vi "ShowRange.Calc.vi"(6 "X-axis devision":i32=1 min=1 max=512, 7 "Current Grating Density":enum16{"150", "300", "600", "1200", "1800"}(ring)=enum."600" caption="Grating Density", 8 "Central Wavelength":dbl=600.0 format="%.2f") -> (0 "meV (Max)":dbl=2170.4007572687524 format="%.2f", 1 "X-axis":dbl[](array[numeric])=[571.2504622529284, 585.6489231225254, 600.0000000000001, 614.300024178551, 628.5453659653462] format="%.4f", 2 "meV (Min)":dbl=1972.5583911666886 format="%.2f", 3 "nm (Max)":dbl=628.5453659653462 format="%.4f", 5 "nm (Min)":dbl=571.2504622529284 format="%.4f")   [LabVIEW 2019]
panel:
  in  "Unit":u16(ring) items=["nm", "cm-1", "meV"]
  out "nm (delta)":dbl=57.29490371241775 format="%.4f"
  out "cm-1 (delta)":dbl=1595.705715333208 format="%.2f"
  out "meV (delta)":dbl=197.8423661020638 format="%.2f"
  out "cm-1 (Max)":dbl=17505.45629418217 format="%.2f"
  out "cm-1 (Min)":dbl=15909.750578848963 format="%.2f"
  out "Detector Pixel Distance":dbl=27.0 format="%.2f"
  out "beta":dbl=0.03851514953863218 format="%.2f"
  out "alpha":dbl=21.141484850461367 format="%.2f"
  out "Spectrometer Mirror angle":dbl=21.18 format="%.2f"
  out "Spectrometer Focal length":dbl=750.0 format="%.1f"
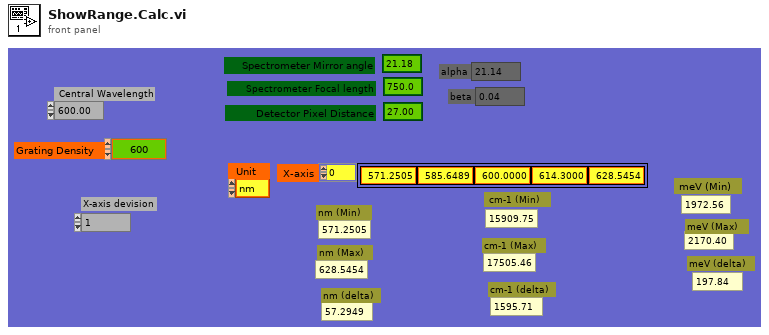
[diagram p1: front panel]
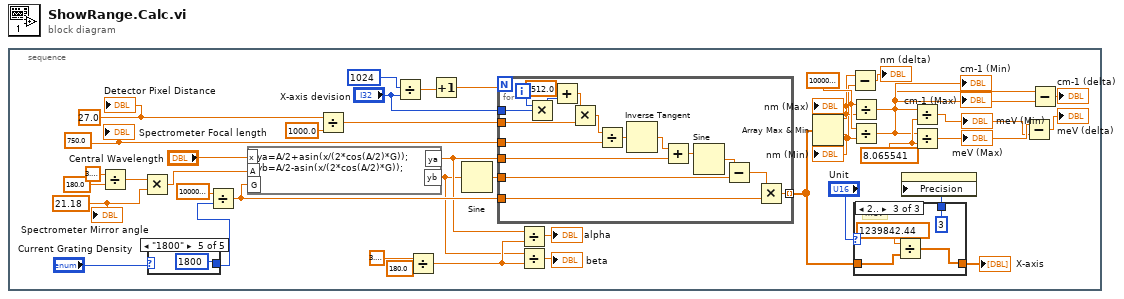
[diagram p0: block diagram]
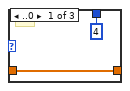
[diagram p2: hidden frame]
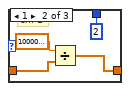
[diagram p3: hidden frame]
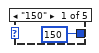
[diagram p4: hidden frame]
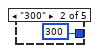
[diagram p5: hidden frame]
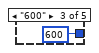
[diagram p6: hidden frame]
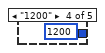
[diagram p7: hidden frame]
diagram:
  n1 = stacked-sequence {
    frame #0 {
      w23 = 21.18 ("Detector Pixel Distance")
      w22 = 750.0 ("Detector Pixel Distance")
      w24 = 27.0 ("x")
      w34 = 8.065541
      w35 = 10000000.0
      n2 = Divide(x=3.141592653589793, y=180.0) -> (x/y=w16:dbl)
      n3 = Multiply(x=w16, y=w23) -> (x*y=w21:dbl)
      n4 = case shown="\"1800\"" "Current Grating Density" {
        tunnel: [150 300 600 1200 1800] -> w10
        frame "150" {
        }
        frame "300" {
        }
        frame "600" {
        }
        frame "1200" {
        }
        frame "1800" {
        }
      }
      n5 = Divide(x=1000000.0, y=w10) -> (x/y=w20:dbl)
      n6 = formula code="ya=A/2+asin(x/(2*cos(A/2)*G));\nyb=A/2-asin(x/(2*cos(A/2)*G));"("x"="Central Wavelength", "A"=w21, "G"=w20) -> ("ya"=w14:dbl, "yb"=w13:dbl)
      n7 = Divide(x=w24, y=1000.0) -> (x/y=w37:dbl)
      n8 = Divide(x=1024, y="X-axis devision") -> (x/y=w2:dbl)
      n9 = Divide(x=3.141592653589793, y=180.0) -> (x/y=w19:dbl)
      n10 = Increment(x=w2) -> (x+1=w1:dbl)
      n11 = Sine(x=w13) -> (sin(x)=w36:dbl)
      n12 = for {
        N: w1 -> [_]
        tunnel: w22 -> [w72]
        tunnel: w37 -> [w61]
        tunnel: w36 -> [w70]
        tunnel: [w68] -> w5 mode=indexing
        tunnel: w20 -> [w67]
        tunnel: w14 -> [w62]
        tunnel: "X-axis devision" -> [w57]
        i -> [w73]
        n13 = Multiply(x=w73, y=w57) -> (x*y=w59:i32)
        n14 = Add(x=-512.0, y=w59) -> (x+y=w58:dbl)
        n15 = Multiply(x=w58, y=w61) -> (x*y=w63:dbl)
        n16 = Divide(x=w63, y=w72) -> (x/y=w66:dbl)
        n17 = Inverse Tangent(1:w66) -> (0:w65:dbl)
        n18 = Add(x=w65, y=w62) -> (x+y=w64:dbl)
        n19 = Sine(x=w64) -> (sin(x)=w71:dbl)
        n20 = Subtract(x=w71, y=w70) -> (x-y=w69:dbl)
        n21 = Multiply(x=w69, y=w67) -> (x*y=w68:dbl)
      }
      n22 = Divide(x=w14, y=w19) -> (x/y=→"alpha":dbl)
      n23 = Divide(x=w13, y=w19) -> (x/y=→"beta":dbl)
      n24 = Array Max & Min(array=w5) -> (max value=w28:dbl, min value=w27:dbl)  [unwired: 2 out]
      "nm (Max)" <- w28
      "nm (Min)" <- w27
      n25 = Subtract(x=w28, y=w27) -> (x-y=→"nm (delta)":dbl)
      n26 = Divide(x=w35, y=w28) -> (x/y=w32:dbl)
      "cm-1 (Min)" <- w32
      n27 = Divide(x=w35, y=w27) -> (x/y=w31:dbl)
      "cm-1 (Max)" <- w31
      n28 = case shown="2.." "Unit" {
        tunnel: w5 -> [w43 w46 w50]
        tunnel: [w43 w45 w49] -> w8
        tunnel: [4 2 3] -> w7
        frame ..0 {
          # "nm"
        }
        frame 1 {
          # "cm-1"
          n29 = Divide(x=10000000.0, y=w46) -> (x/y=w45:dbl[])
        }
        frame 2.. {
          # "meV"
          n30 = Divide(x=1239842.44, y=w50) -> (x/y=w49:dbl[])
        }
      }
      "X-axis" <- w8
      n31 = property class="DigNum (strict)"("Precision"=w7) -> ()  [unwired: 2 in, 2 out]
      n32 = Divide(x=w32, y=w34) -> (x/y=w30:dbl)
      "meV (Min)" <- w30
      n33 = Divide(x=w31, y=w34) -> (x/y=w33:dbl)
      "meV (Max)" <- w33
      n34 = Subtract(x=w33, y=w30) -> (x-y=→"meV (delta)":dbl)
      n35 = Subtract(x=w31, y=w32) -> (x-y=→"cm-1 (delta)":dbl)
      "Spectrometer Focal length" <- w22
      "Spectrometer Mirror angle" <- w23
      "Detector Pixel Distance" <- w24
    }
  }
